vi "ExSubPullStrip.vi"(3 "error in (no error)":errorcluster, 4 "Strip to pull out":u32, 5 "Image Handle":u32) -> (0 "error out":errorcluster, 1 "New Image Handle":u32, 2 "Image handle":u32)   [LabVIEW 2010]
panel:
  # "ExSubPullStrip.vi : this subroutine pulls a strip out of a frame and \nand generates a new image handle of the same x dimension of \nprevious frame but only made up of the specified strip."
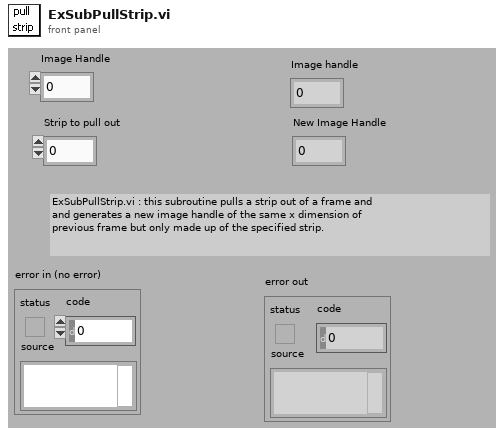
[diagram p1: front panel]
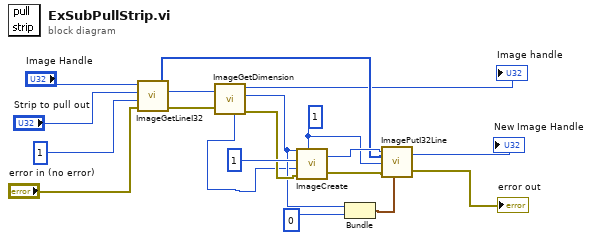
[diagram p0: block diagram]
diagram:
  w9 = 1
  n1 = call <userlib>:"ImageGetLineI32.vi"("error in"="error in (no error)", "Z Position"=1, "Y Position"="Strip to pull out", "Data Handle"="Image Handle") -> ("error out"=w14:errorcluster, "Array i32"=w10:i32[], "Data Handle"=w15:u32)
  n2 = call <userlib>:"ImageGetDimension.vi"("Image Handle"=w15, "error in"=w14) -> ("Data type"=w1:u32, "Image Handle"=→"Image handle":u32, "X dimension"=w7:u32, "error out"=w12:errorcluster)  [unwired: 2 out]
  n3 = call <userlib>:"ImageCreate.vi"("X dimension"=w7, "Y dimension"=1, "Data Type"=w1, "error in"=w12, "Number Of Frames"=w9) -> ("Image Handle"=w11:u32, "error out"=w8:errorcluster)
  n4 = Bundle("X dimension"=w7, 0) -> (w5:cluster{"X dimension":u32, i32})  [unwired: 1 in]
  n5 = call <userlib>:"ImagePutI32Line.vi"("Image Handle"=w11, "Image Data"=w10, "Y Position"=w9, "error in (no error)"=w8, "Image dimensions"=w5) -> ("Image Handle"=→"New Image Handle":u32, "error out"=→"error out":errorcluster)
